vi "ProjectVersionCheck_Provider_Interface.vi"() -> (3 "Interface Table":T1)   [LabVIEW 2015]
uses:
  <resource>/Framework/Providers/API/Provider_Interface.ctl
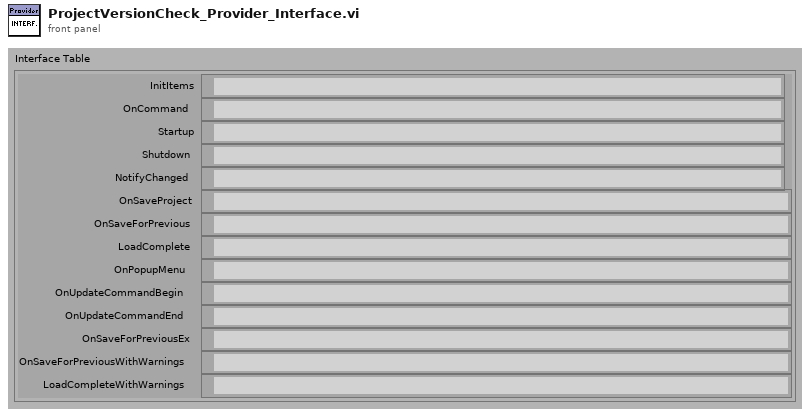
[diagram p1: front panel]
types:
  T1 = typedef "Provider_Interface.ctl" = cluster{"InitItems":path, "OnCommand":path, "Startup":path, "Shutdown":path, "NotifyChanged":path, "OnSaveProject":path, "OnSaveForPrevious":path, "LoadComplete":path, "OnPopupMenu":path, "OnUpdateCommandBegin":path, "OnUpdateCommandEnd":path, "OnSaveForPreviousEx":path, "OnSaveForPreviousWithWarnings":path, "LoadCompleteWithWarnings":path}
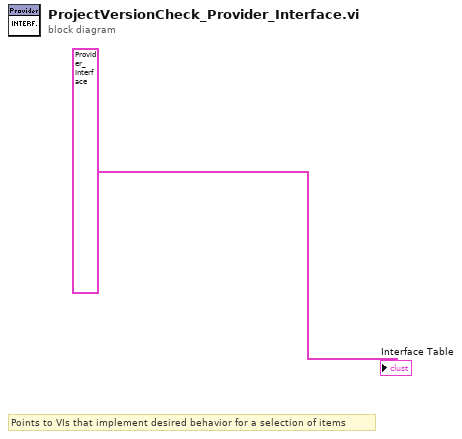
[diagram p0: block diagram]
diagram:
  # "Points to VIs that implement desired behavior for a selection of items"
  "Interface Table" <- T1 {"InitItems"=path "", "OnCommand"=path "", "Startup"=path "", "Shutdown"=path "", "NotifyChanged"=path "", "OnSaveProject"=path "", "OnSaveForPrevious"=path "", "LoadComplete"=path "", "OnPopupMenu"=path "", "OnUpdateCommandBegin"=path "", "OnUpdateCommandEnd"=path "", "OnSaveForPreviousEx"=path "", "OnSaveForPreviousWithWarnings"=path "", "LoadCompleteWithWarnings"=path ""} ("InterfaceTable")
